vi "offset calculator.vi"(11 "offset":T2) -> (3 "Tool Offsets":T1)   [LabVIEW 2016]
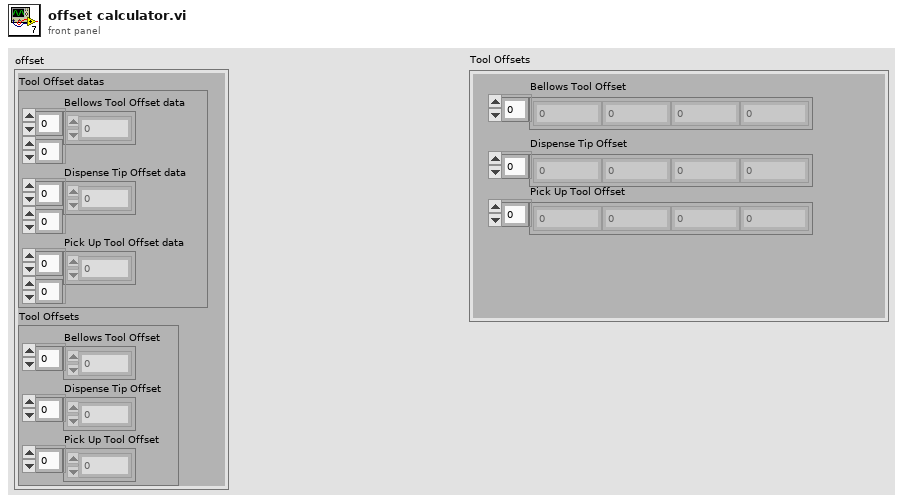
[diagram p1: front panel]
types:
  T1 = cluster{"Bellows Tool Offset":dbl[], "Dispense Tip Offset":dbl[], "Pick Up Tool Offset":dbl[]}
  T2 = cluster{"Tool Offset datas":cluster{"Bellows Tool Offset data":dbl[][], "Dispense Tip Offset data":dbl[][], "Pick Up Tool Offset data":dbl[][]}, "Tool Offsets":cluster{"Bellows Tool Offset":dbl[], "Dispense Tip Offset":dbl[], "Pick Up Tool Offset":dbl[]}}
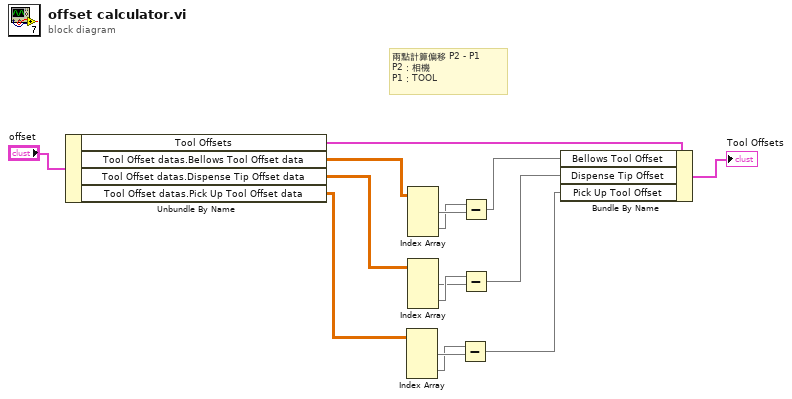
[diagram p0: block diagram]
diagram:
  # "兩點計算偏移 P2 - P1\nP2：相機 \nP1：TOOL"
  n1 = Unbundle By Name("offset") -> ("Tool Offsets"=w13:T1, "Tool Offset datas.Bellows Tool Offset data"=w5:dbl[][], "Tool Offset datas.Dispense Tip Offset data"=w4:dbl[][], "Tool Offset datas.Pick Up Tool Offset data"=w12:dbl[][])
  n2 = Index Array(array=w12) -> (element #1=w11:dbl[], element #2=w10:dbl[])  [unwired: 4 in]
  n3 = Index Array(array=w5) -> (element #1=w7:dbl[], element #2=w6:dbl[])  [unwired: 4 in]
  n4 = Index Array(array=w4) -> (element #1=w8:dbl[], element #2=w9:dbl[])  [unwired: 4 in]
  n5 = Subtract(x=w10, y=w11) -> (x-y=w3:dbl[])
  n6 = Subtract(x=w6, y=w7) -> (x-y=w1:dbl[])
  n7 = Subtract(x=w9, y=w8) -> (x-y=w2:dbl[])
  n8 = Bundle By Name(cluster=w13, "Bellows Tool Offset"=w1, "Dispense Tip Offset"=w2, "Pick Up Tool Offset"=w3) -> (→"Tool Offsets":T1)
